vi "Move Needle.vi"(8 "error in (no error)":errorcluster, 10 "Needle Position":T1, 11 "Autosampler in":refnum<class "Autosampler.lvclass">) -> (0 "error out":errorcluster, 3 "Autosampler out":refnum<class "Autosampler.lvclass">)   [LabVIEW 2023, in "Autosampler.lvlib" / "Autosampler.lvclass"]
uses:
  Autosampler.lvclass
  Autosampler Needle Position.ctl
  Autosampler.lvclass/Autosampler.ctl
  Autosampler State2.ctl
  Autosampler.lvlib
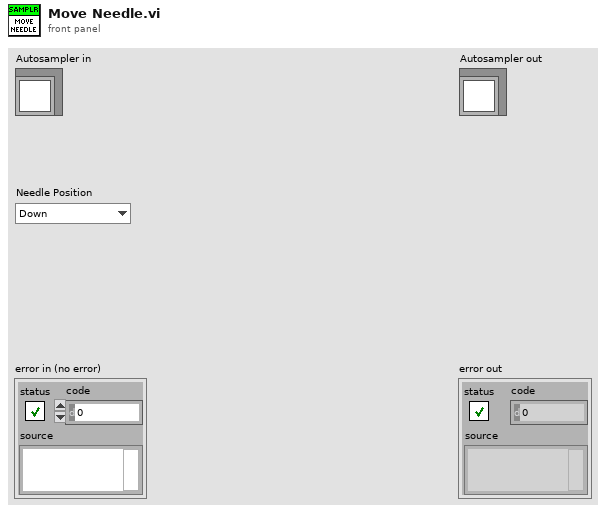
[diagram p1: front panel]
types:
  T1 = typedef "Autosampler.lvlib/Autosampler Needle Position.ctl" = enum16{"Down", "Up"}
  T2 = typedef "Autosampler.lvlib/Autosampler State2.ctl" = enum16{"Error", "Idle", "Positioning", "Pumping", "Shaking", "Washing", "Priming"}
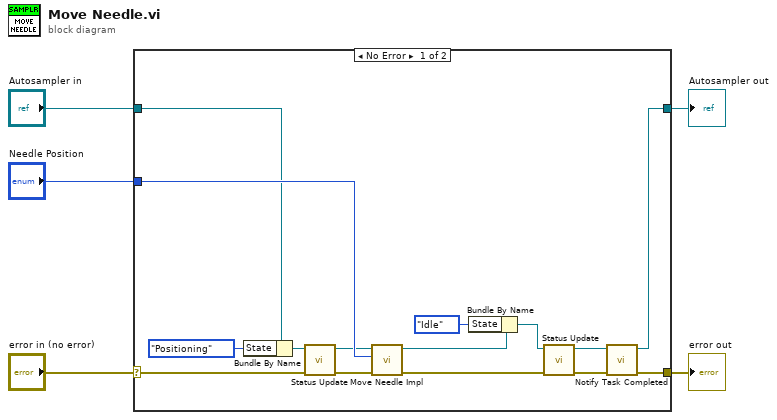
[diagram p0: block diagram]
diagram:
  n1 = case shown="No Error" "error in (no error)" {
    selector: "error in (no error)" -> [w14 w22]
    tunnel: [w18 w22] -> w4
    tunnel: [w17 w21] -> w2
    tunnel: "Autosampler in" -> [w11 w21]
    tunnel: "Needle Position" -> [w15 _]
    frame No Error {
      n2 = Bundle By Name(cluster=w11, "State"=Autosampler_State2."Positioning") -> (w12:refnum<class "Autosampler.lvclass">)
      n3 = call "Status Update.vi"("error in (no error)"=w14, "Autosampler in"=w12) -> ("error out"=w13:errorcluster, "Autosampler out"=w9:refnum<class "Autosampler.lvclass">)  [unwired: 7 in, 1 out]
      n4 = call-dynamic "Move Needle Impl.vi"("error in (no error)"=w13, "Needle Position"=w15, "Autosampler in"=w9) -> ("error out"=w16:errorcluster, "Autosampler out"=w6:refnum<class "Autosampler.lvclass">)  [unwired: 7 in]
      n5 = Bundle By Name(cluster=w6, "State"=Autosampler_State2."Idle") -> (w7:refnum<class "Autosampler.lvclass">)
      n6 = call "Status Update.vi"("error in (no error)"=w16, "Autosampler in"=w7) -> ("error out"=w19:errorcluster, "Autosampler out"=w20:refnum<class "Autosampler.lvclass">)  [unwired: 7 in, 1 out]
      n7 = call-dynamic "Notify Task Completed.vi"("error in (no error)"=w19, "Device in"=w20) -> ("error out"=w18:errorcluster, "Device out"=w17:refnum<class "Autosampler.lvclass">)  [unwired: 8 in]
    }
    frame Error {
    }
  }
  "error out" <- w4
  "Autosampler out" <- w2
